vi "ScpiGetHandle.vi"(7 "error in (no error)":errorcluster, 9 "TCP port":u16=5025 min=1025 step=1, 10 "IP Address":string="localhost") -> (0 "Error out":errorcluster, 3 "connection ID":refnum<k5>)   [LabVIEW 2009]
doc: "Sends a SCPI command to an instrument.\nWaits for the reply.\nReply string must end in NewLine character.\nFirst, get the \"handle\" or TCP connection ID"
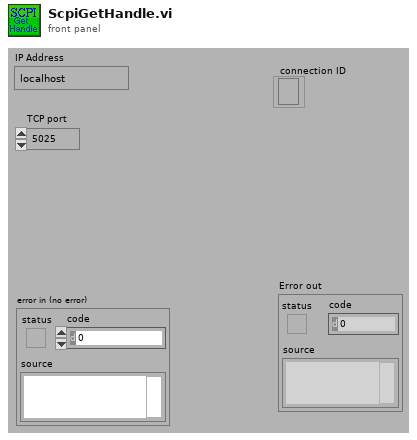
[diagram p1: front panel]
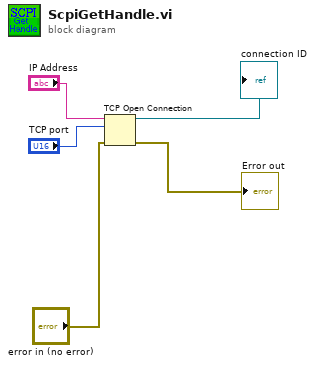
[diagram p0: block diagram]
diagram:
  n1 = TCP Open Connection(address="IP Address", remote port or service name="TCP port", error in (no error)="error in (no error)") -> (connection ID=→"connection ID":refnum<k5>, error out=→"Error out":errorcluster)  [unwired: 2 in]
